vi "UART Init Device.vi"(7 "pInitConfig":T1, 9 "UARTIndex":i32, 10 "DevIndex":i32, 11 "DevType":i32) -> (3 "function return":i32, 5 "pInitConfig out":T1)   [LabVIEW 2010, in "ControlUART.lvlib"]
doc: "int WINAPI UART_InitDevice(int DevType,int DevIndex,int UARTIndex, PUART_INIT_CONFIG pInitConfig);"
uses:
  ControlUART.lvlib
  ControlUART/Ginkgo_Driver.dll
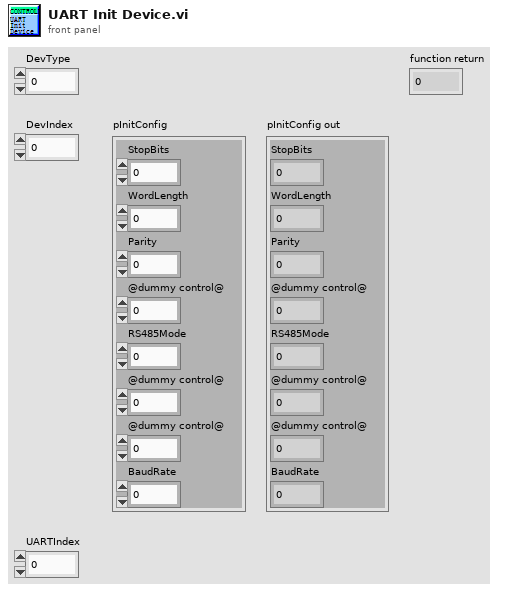
[diagram p1: front panel]
types:
  T1 = cluster{"StopBits":u8, "WordLength":u8, "Parity":u8, "@dummy control@":i8, "RS485Mode":u16, "@dummy control@":i8, "@dummy control@":i8, "BaudRate":u32}
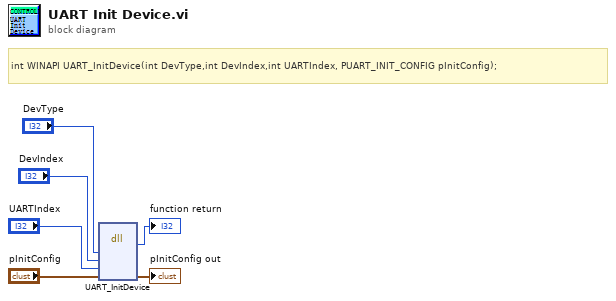
[diagram p0: block diagram]
diagram:
  # "int WINAPI UART_InitDevice(int DevType,int DevIndex,int UARTIndex, PUART_INIT_CONFIG pInitConfig);"
  n1 = dll-call lib="E:/Project/vt_ginkgo/truck/Ginkgo Driver/vs2010/Ginkgo_USB-I2C&SPI&CAN_API_v2.0.3.3/lib/labview_32bit/ControlUART/Ginkgo_Driver.*" fn="UART_InitDevice"("DevType"="DevType", "DevIndex"="DevIndex", "UARTIndex"="UARTIndex", "pInitConfig"="pInitConfig") -> (→"function return":i32, "pInitConfig"=→"pInitConfig out":T1)  [unwired: 6 in, 2 out]
